vi "Set Advanced Trigger Mode State.vi"(11 "iState":i32) -> (3 "function return":u32)   [LabVIEW 2018, in "Copy of Andor SDK.lvlib"]
doc: "EXPNETTYPE unsigned int WINAPI SetAdvancedTriggerModeState(int iState);"
uses:
  Copy of Andor SDK.lvlib
  <userlib>/Andor SDK/ATMCD32D.dll
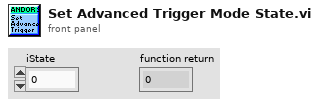
[diagram p1: front panel]
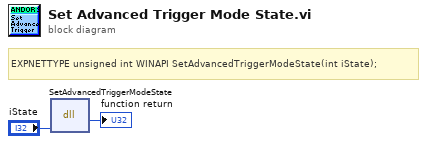
[diagram p0: block diagram]
diagram:
  # "EXPNETTYPE unsigned int WINAPI SetAdvancedTriggerModeState(int iState);"
  n1 = dll-call lib="C:/Program Files (x86)/National Instruments/LabVIEW 2018/user.lib/Andor SDK/ATMCD32D.*" fn="SetAdvancedTriggerModeState"("iState"="iState") -> (→"function return":u32)  [unwired: 4 in, 2 out]
